vi "ImagesToInlineHTML.vi"(10 "attachmentsIn":path[](array[path])) -> (1 "inlinedAttachments":path[](array[path]), 2 "remainingAttachments":path[](array[path]), 4 "HTMLimgs":string)   [LabVIEW 2022 SP3]
panel:
  # "base64 encodes gif, jpg and png images and wraps in HTML to allow inline display in emails"
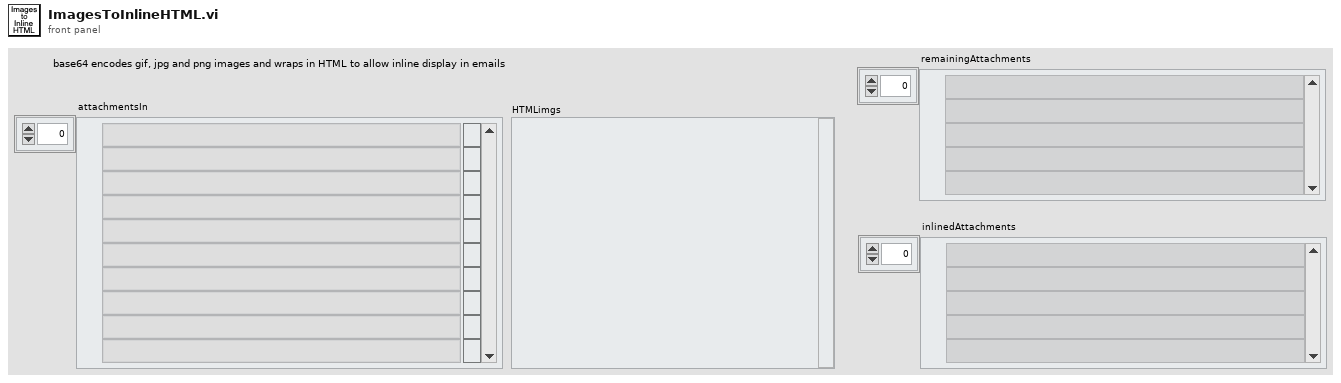
[diagram p1: front panel]
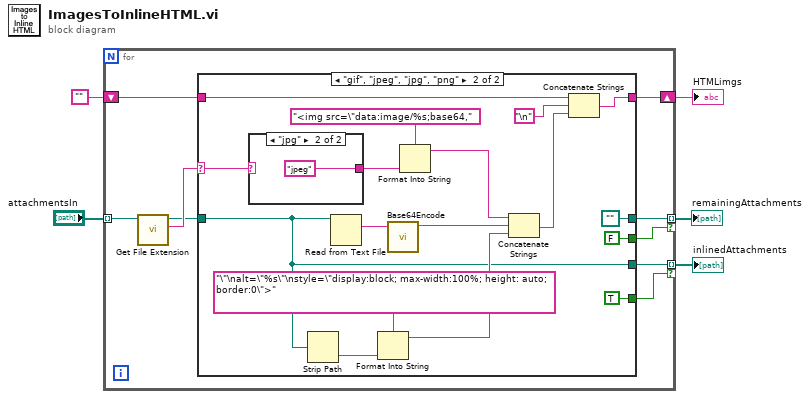
[diagram p0: block diagram]
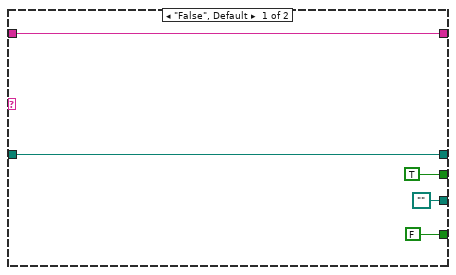
[diagram p2: hidden frame]
diagram:
  n1 = for {
    tunnel: "attachmentsIn" -> [w6] mode=indexing
    shift-right: [w14] -> w4
    shift-left: "" -> [w13]
    tunnel: [w11] -> w1 mode=indexing if=w9
    tunnel: [w10] -> w2 mode=indexing if=w8
    n2 = call <vilib>:"Get File Extension.vi"("file"=w6) -> ("lowercase file extension"=w12:string, "dup file"=w7:path)  [unwired: 6 in, 3 out]
    n3 = case shown="\"gif\", \"jpeg\", \"jpg\", \"png\"" w12 {
      selector: w12 -> [_ w26]
      tunnel: [w19 w32] -> w14
      tunnel: w13 -> [w19 w31]
      tunnel: w7 -> [w18 w21]
      tunnel: [path "" ("path") w21] -> w11
      tunnel: [w18 path "" ("path")] -> w10
      tunnel: [FALSE TRUE] -> w9
      tunnel: [TRUE FALSE] -> w8
      frame "False", Default {
      }
      frame "gif", "jpeg", "jpg", "png" {
        n4 = case shown="\"jpg\"" w26 {
          selector: w26 -> [w37 _]
          tunnel: [w37 "jpeg"] -> w25
          frame "False", Default {
          }
          frame "jpg" {
          }
        }
        n5 = Strip Path(path=w21) -> (name=w20:string)  [unwired: 1 out]
        n6 = Read from Text File(file (use dialog)=w21) -> (text=w36:string)  [unwired: 3 in, 3 out]
        n7 = Format Into String(format string="\"\nalt=\"%s\"\nstyle=\"display:block; max-width:100%; height: auto; border:0\">" ("postString"), w20) -> (resulting string=w29:string)  [unwired: 2 in, 1 out]
        n8 = call "Base64Encode.vi"("String"=w36) -> ("Base64 String"=w35:string)  [unwired: 10 in]
        n9 = Format Into String(format string="<img src=\"data:image/%s;base64," ("preString"), w25) -> (resulting string=w27:string)  [unwired: 2 in, 1 out]
        n10 = Concatenate Strings(w27, w35, w29) -> (w33:string)
        n11 = Concatenate Strings(w31, "\n", w33) -> (w32:string)
      }
    }
  }
  "HTMLimgs" <- w4
  "inlinedAttachments" <- w1
  "remainingAttachments" <- w2
